vi "PixelClockU32.vi"(10 "Samples per pixel":u32=16960, 11 "Sample counter":u32=16960) -> (3 "Pixel clock":bool)   [LabVIEW 2012]
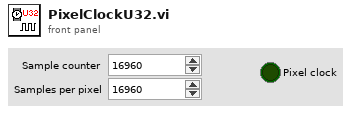
[diagram p1: front panel]
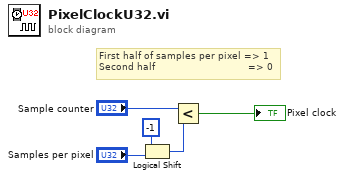
[diagram p0: block diagram]
diagram:
  # "First half of samples per pixel => 1\nSecond half                               => 0"
  n1 = Logical Shift(y=i16 -1, x="Samples per pixel") -> (x << y=w2:u32)
  n2 = Less?(x="Sample counter", y=w2) -> (x < y?=→"Pixel clock":bool)
